vi "Configure.vi"(8 "error in (no error)":errorcluster, 10 "Preceding Items":refnum<class "Item.lvclass">[](array[class]), 11 "ZIP Item in":refnum<class "ZIP Item.lvclass">) -> (0 "error out":errorcluster, 3 "ZIP Item out":refnum<class "ZIP Item.lvclass">)   [LabVIEW 2019, in "ZIP.lvlib" / "ZIP Item.lvclass"]
uses:
  ZIP Item.lvclass
  libs/Solution.lvlibp/Solution/Item/Item.lvclass
  ZIP Item.lvclass/ZIP Item.ctl
panel:
  in  "File Path":path
  in  "OK":bool
  in  "Cancel":bool
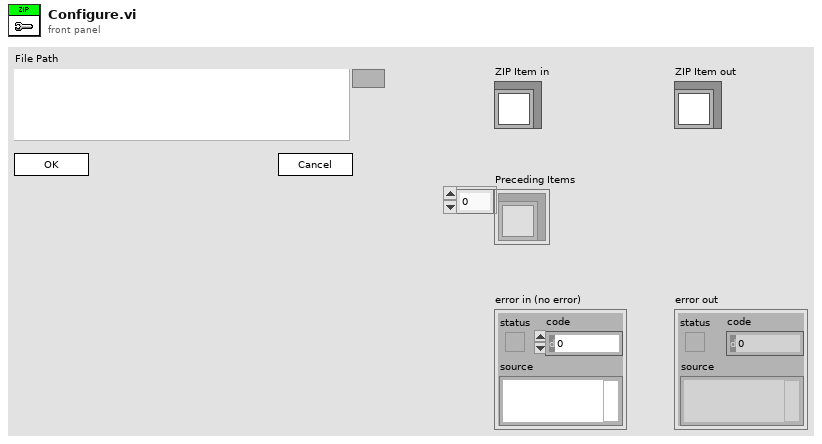
[diagram p1: front panel]
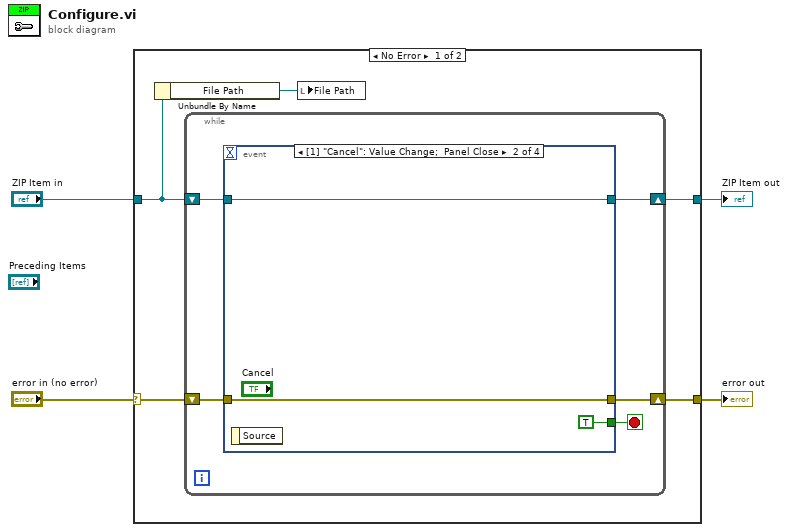
[diagram p0: block diagram]
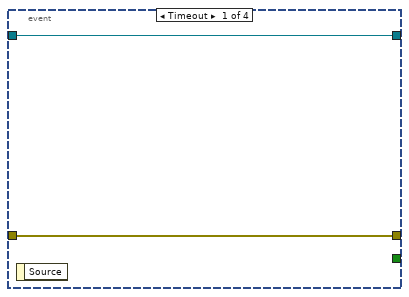
[diagram p2: hidden frame]
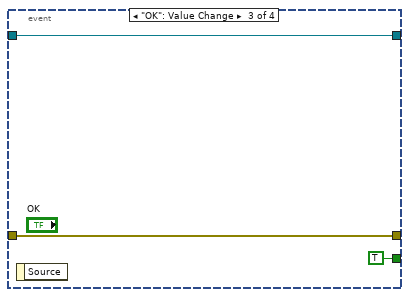
[diagram p3: hidden frame]
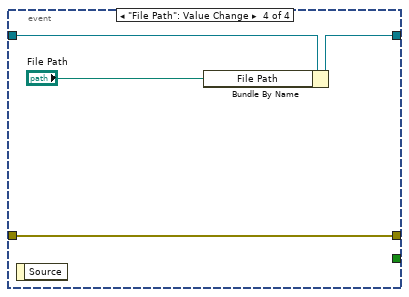
[diagram p4: hidden frame]
diagram:
  n1 = case shown="No Error" "error in (no error)" {
    selector: "error in (no error)" -> [w7 w28]
    tunnel: [w8 w28] -> w3
    tunnel: [w9 w27] -> w1
    tunnel: "ZIP Item in" -> [w6 w27]
    frame No Error {
      n2 = Unbundle By Name(w6) -> ("File Path"=w5:path)
      n3 = while {
        shift-right: [w13] -> w8
        shift-left: w7 -> [w12]
        shift-right: [w14] -> w9
        shift-left: w6 -> [w11]
        stop <- w10 stop-if-true
        n4 = event shown="[1] \"Cancel\": Value Change;  Panel Close" {
          selector: _ -> [_ _ _ _]
          dyn-events: _ -> [_ _ _ _]
          timeout: _ -> [_ _ _ _]
          tunnel: w11 -> [w16 w19 w22 w26]
          tunnel: [w16 w19 w22 w24] -> w14
          tunnel: [w15 w18 w21 w25] -> w13
          tunnel: w12 -> [w15 w18 w21 w25]
          tunnel: [_ TRUE TRUE _] -> w10
          event Timeout {
            n5 = event-data() -> ()  [unwired: 1 in, 1 out]
          }
          event "Cancel": Value Change; Panel Close {
            n6 = event-data() -> ()  [unwired: 1 in, 1 out]
          }
          event "OK": Value Change {
            n7 = event-data() -> ()  [unwired: 1 in, 1 out]
          }
          event "File Path": Value Change {
            n8 = event-data() -> ()  [unwired: 1 in, 1 out]
            n9 = Bundle By Name(cluster=w26, "File Path"="File Path") -> (w24:refnum<class "ZIP Item.lvclass">)
          }
        }
      }
      n10 = local write "File Path"(w5) -> ()
    }
    frame Error {
    }
  }
  "error out" <- w3
  "ZIP Item out" <- w1
